vi "ActionVIOnRecompile.vi"(8 "error in":errorcluster, 9 "Timeout (ms)":u32, 10 "Runtime Configurable Section Path":string, 11 "Device Item Ref in":T1 format="%.0x") -> (0 "error out":errorcluster)   [LabVIEW 2026, in "Runtime Configuration Support Inline Async Example Custom Device System Explorer.lvlib"]
uses:
  Runtime Configuration Support Inline Async Example Custom Device System Explorer.lvlib
  <vilib>/NI VeriStand/Custom Device API/Custom Device Item Ref.ctl
  <vilib>/NI VeriStand/Custom Device API/Custom Device Channel Type.ctl
  <vilib>/NI VeriStand/Custom Device API/Block Data Reference.ctl
  <vilib>/NI VeriStand/Custom Device API/Data Reference.ctl
  Shared/Reconfigured.Settings.ctl
  Shared/Compiled.Settings.ctl
  <vilib>/NI VeriStand/Custom Device API/Get Item Property (I32).vi
  Error Constants.vi
  <vilib>/NI VeriStand/Custom Device API/Get Item Property (Variant).vi
  <vilib>/NI VeriStand/Execution/CustomDevice/NI VeriStand - Send Custom Device Message (Byte Array).vi
  <vilib>/NI VeriStand/Custom Device API/Custom Device API.lvlib
  <vilib>/NI/NIVS Inline Async API/_Data Access System Explorer/Data Access System Explorer.lvlib
  <vilib>/NI VeriStand/execution/CustomDevice/NI_VS Custom Device ExecutionAPI.lvlib
  Shared/Runtime Configuration Support Inline Async Example Custom Device Shared.lvlib
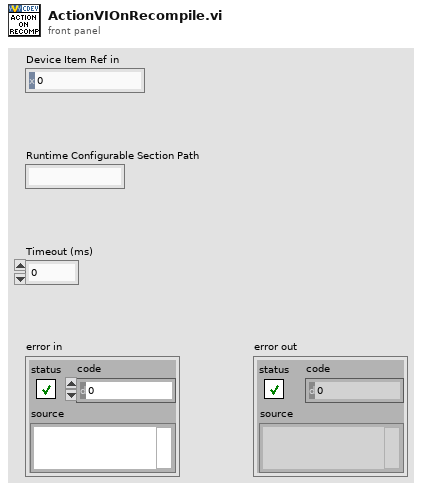
[diagram p1: front panel]
types:
  T1 = typedef "Custom Device API.lvlib/Custom Device Item Ref.ctl" = u64
  T2 = typedef "Runtime Configuration Support Inline Async Example Custom Device Shared.lvlib/Reconfigured.Settings.ctl" = cluster{"Compiled.Settings":T3, "Compiled Inline Async Settings":cluster{"Read":cluster{"Refs":T4[], "Values":dbl[]}[], "Write":cluster{"Refs":T4[], "Values":dbl[]}[], "ReadWrite":cluster{"Refs":T5[], "Values":dbl[], "Reset Values":dbl[]}[], "LUT":variant}, "Response Ref":refnum<queue>}
  T3 = typedef "Runtime Configuration Support Inline Async Example Custom Device Shared.lvlib/Compiled.Settings.ctl" = cluster{"Name":string, "Async Init Timeout":u16, "Inport SignalIDs":i32[], "Outport SignalIDs":i32[], "Inport Values":dbl[], "Outport Values":dbl[], "Dynamic Config Status":bool, "Device Error":errorcluster}
  T4 = typedef "Custom Device API.lvlib/Block Data Reference.ctl" = cluster{"Data Reference":T5, "Offset":u64, "Length":u64}
  T5 = typedef "Custom Device API.lvlib/Data Reference.ctl" = i32
  T6 = typedef "Custom Device API.lvlib/Custom Device Channel Type.ctl" = enum16{"Input", "Output"}
  T7 = cluster{"Name":string, "Type":enum16{"Output/Write", "Input/Read", "Input/ReadWrite"}, "VS Refs":T1[]}
  T8 = enum16{"Output/Write", "Input/Read", "Input/ReadWrite"}
  T9 = cluster{"Read":cluster{"Refs":T4[], "Values":dbl[]}[], "Write":cluster{"Refs":T4[], "Values":dbl[]}[], "ReadWrite":cluster{"Refs":T5[], "Values":dbl[], "Reset Values":dbl[]}[], "LUT":variant}
  T10 = typedef "Custom Device API.lvlib/Custom Device Item Info.ctl" = cluster{"Name":string, "Is Channel":bool, "GUID":string, "Is Waveform":bool}
  T11 = cluster{"Name":string, "Type":enum16{"Output/Write", "Input/Read", "Input/ReadWrite"}, "VS Refs":T1[]}[]
  T12 = typedef "NI_VS Custom Device ExecutionAPI.lvlib/Custom Device Ref.ctl" = refnum<k24>
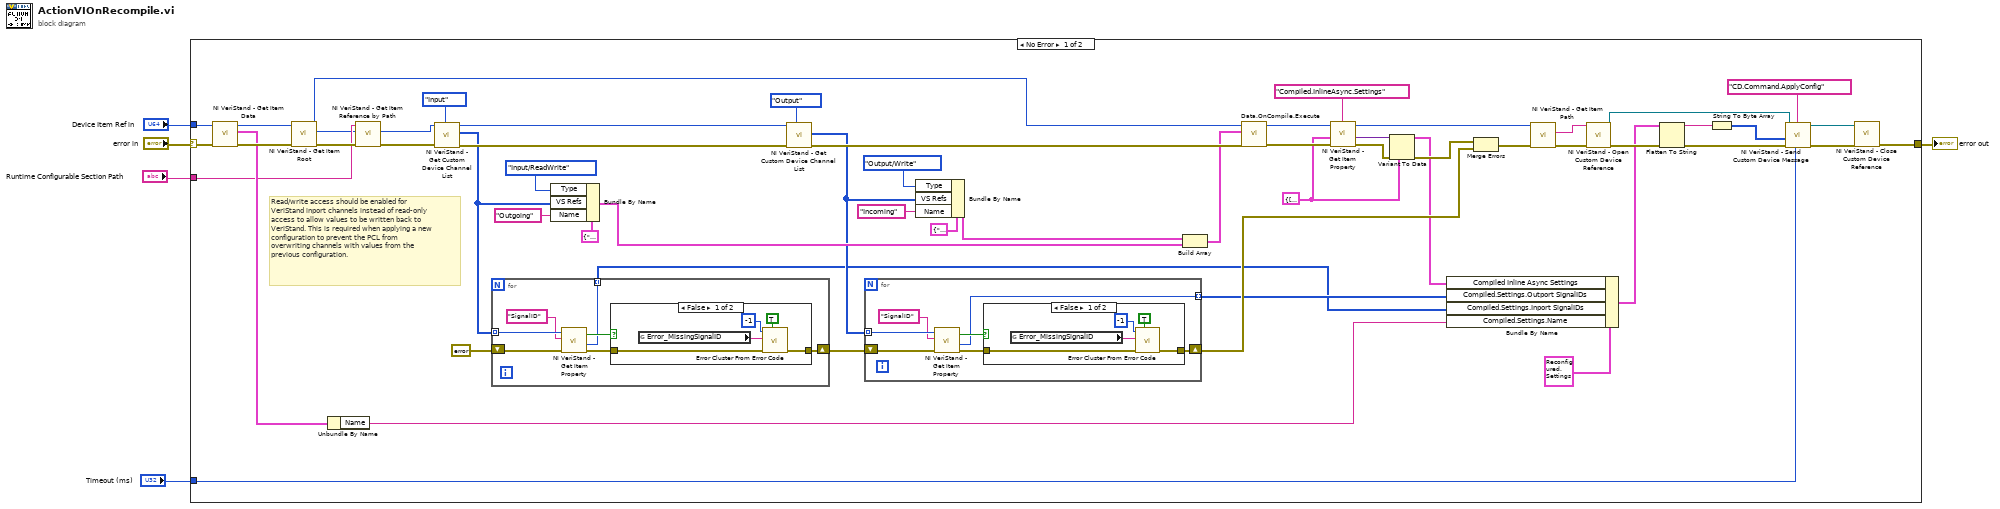
[diagram p0: block diagram]
diagram:
  n1 = case shown="No Error" "error in" {
    selector: "error in" -> [w62 w89]
    tunnel: [w54 w89] -> w4
    tunnel: "Device Item Ref in" -> [w44 _]
    tunnel: "Runtime Configurable Section Path" -> [w32 _]
    tunnel: "Timeout (ms)" -> [w17 _]
    frame No Error {
      w15 = T9 {"Read"=[], "Write"=[], "ReadWrite"=[], "LUT"=variant} ("Compiled.InlineAsync.Settings")
      # "Read/write access should be enabled for VeriStand inport channels instead of read-only access to allow values to be written back to VeriStand. This is required when applying a new configuration to prevent the PCL from overwriting channels with values from the previous configuration."
      n2 = call <vilib>:"NI VeriStand - Get Item Data.vi"("error in (no error)"=w62, "Item Ref in"=w44) -> ("error out"=w46:errorcluster, "Item Info"=w43:T10, "Item Ref out"=w8:T1)  [unwired: 6 in, 1 out]
      n3 = call <vilib>:"NI VeriStand - Get Item Root.vi"("error in (no error)"=w46, "Item Ref in"=w8) -> ("error out"=w45:errorcluster, "Root Ref out"=w9:T1, "Item Ref out"=w7:T1)  [unwired: 6 in, 1 out]
      n4 = Unbundle By Name(w43) -> ("Name"=w42:string)
      n5 = call <vilib>:"NI VeriStand - Get Item Reference by Path.vi"("error in (no error)"=w45, "Root Ref"=w9, "Item Path in"=w32) -> ("error out"=w61:errorcluster, "Item Ref"=w31:T1)  [unwired: 5 in, 2 out]
      n6 = call <vilib>:"NI VeriStand - Get Custom Device Channel List.vi"("Channel Type"=Custom_Device_Channel_Type."Input", "error in (no error)"=w61, "Device Ref in"=w31) -> ("error out"=w60:errorcluster, "Specified Channel Ref List"=w14:T1[], "Device Ref out"=w28:T1)  [unwired: 6 in]
      n7 = for {
        tunnel: w14 -> [w79] mode=indexing
        shift-right: [w81] -> w50
        shift-left: errorcluster {"status"=FALSE, "code"=0, "source"=""} ("error out") -> [w80]
        tunnel: [w76] -> w10 mode=indexing
        n8 = call-poly <vilib>:"NI VeriStand - Get Item Property.vi"("error in (no error)"=w80, "Property Name"="SignalID", "Item Ref in"=w79) -> ("error out"=w82:errorcluster, "Value"=w76:i32, "Found?"=w77:bool)  [unwired: 5 in, 1 out]
        n9 = case shown="False" w77 {
          tunnel: w82 -> [w87 w88]
          tunnel: [w86 w88] -> w81
          frame False {
            n10 = global read "Error Constants.vi" "Error_MissingSignalID"() -> (w84:string)
            n11 = call <vilib>:"Error Cluster From Error Code.vi"("show call chain? (False)"=TRUE, "error in (no error)"=w87, "error message (\"\")"=w84, "error code (0)"=-1) -> ("error out"=w86:errorcluster)  [unwired: 5 in]
          }
          frame True {
          }
        }
      }
      n12 = Bundle By Name(cluster=T7 {"Name"="", "Type"=enum."Output/Write", "VS Refs"=[]} ("Group"), "Type"=T8."Input/ReadWrite", "VS Refs"=w14, "Name"="Outgoing" ("Item Name")) -> (w33:T7)
      n13 = call <vilib>:"NI VeriStand - Get Custom Device Channel List.vi"("Channel Type"=Custom_Device_Channel_Type."Output", "error in (no error)"=w60, "Device Ref in"=w28) -> ("error out"=w59:errorcluster, "Specified Channel Ref List"=w13:T1[])  [unwired: 6 in, 1 out]
      n14 = for {
        tunnel: w13 -> [w66] mode=indexing
        shift-right: [w68] -> w47
        shift-left: w50 -> [w67]
        tunnel: [w63] -> w11 mode=indexing
        n15 = call-poly <vilib>:"NI VeriStand - Get Item Property.vi"("error in (no error)"=w67, "Property Name"="SignalID", "Item Ref in"=w66) -> ("error out"=w69:errorcluster, "Value"=w63:i32, "Found?"=w64:bool)  [unwired: 5 in, 1 out]
        n16 = case shown="False" w64 {
          tunnel: w69 -> [w74 w75]
          tunnel: [w73 w75] -> w68
          frame False {
            n17 = global read "Error Constants.vi" "Error_MissingSignalID"() -> (w71:string)
            n18 = call <vilib>:"Error Cluster From Error Code.vi"("show call chain? (False)"=TRUE, "error in (no error)"=w74, "error message (\"\")"=w71, "error code (0)"=-1) -> ("error out"=w73:errorcluster)  [unwired: 5 in]
          }
          frame True {
          }
        }
      }
      n19 = Bundle By Name(cluster=T7 {"Name"="", "Type"=enum."Output/Write", "VS Refs"=[]} ("Group"), "Type"=T8."Output/Write", "VS Refs"=w13, "Name"="Incoming" ("Item Name")) -> (w38:T7)
      n20 = Build Array(w38, w33) -> (w36:T11)
      n21 = call <vilib>:"Data.OnCompile.Execute.vi"("error in"=w59, "VS Ref Groups"=w36, "Custom Device Ref"=w7) -> ("error out"=w57:errorcluster, "Custom Device Ref"=w24:T1)  [unwired: 7 in]
      n22 = call-poly <vilib>:"NI VeriStand - Get Item Property.vi"("error in (no error)"=w57, "Default Value"=w15, "Property Name"="Compiled.InlineAsync.Settings", "Item Ref in"=w24) -> ("error out"=w52:errorcluster, "Value"=w22:variant, "Item Ref out"=w16:T1)  [unwired: 4 in, 1 out]
      n23 = Variant To Data(error in=w52, type=w15, Variant=w22) -> (data=w12:T9, error out=w49:errorcluster)
      n24 = Bundle By Name(cluster=T2 {"Compiled.Settings"={"Name"="", "Async Init Timeout"=0, "Inport SignalIDs"=[], "Outport SignalIDs"=[], "Inport Values"=[], "Outport Values"=[], "Dynamic Config Status"=FALSE, "Device Error"={"status"=FALSE, "code"=0, "source"=""}}, "Compiled Inline Async Settings"={"Read"=[], "Write"=[], "ReadWrite"=[], "LUT"=variant}, "Response Ref"=refnum} ("ReConfigured.Settings"), "Compiled Inline Async Settings"=w12, "Compiled.Settings.Outport SignalIDs"=w11, "Compiled.Settings.Inport SignalIDs"=w10, "Compiled.Settings.Name"=w42) -> (w21:T2)
      n25 = Merge Errors(w49, w47) -> (w48:errorcluster)
      n26 = call <vilib>:"NI VeriStand - Get Item Path.vi"("error in (no error)"=w48, "Item Ref in"=w16) -> ("error out"=w58:errorcluster, "Path"=w27:string)  [unwired: 6 in, 2 out]
      n27 = call <vilib>:"NI VeriStand - Open Custom Device Reference.vi"("error in (no error)"=w58, "Custom Device Path"=w27) -> ("error out"=w56:errorcluster, "Custom Device"=w26:T12)  [unwired: 8 in]
      n28 = Flatten To String(anything=w21, error in (no error)=w56) -> (data string=w20:string, error out=w55:errorcluster)  [unwired: 2 in, 1 out]
      n29 = String To Byte Array(string=w20) -> (unsigned byte array=w19:u8[])
      n30 = call-poly <vilib>:"NI VeriStand - Send Custom Device Message.vi"("Timeout ms (5000)"=w17, "error in (no error)"=w55, "Data"=w19, "Command"="CD.Command.ApplyConfig", "Custom Device in"=w26) -> ("error out"=w53:errorcluster, "Custom Device out"=w18:T12)  [unwired: 4 in, 1 out]
      n31 = call <vilib>:"NI VeriStand - Close Custom Device Reference.vi"("error in (no error)"=w53, "Custom Device"=w18) -> ("error out"=w54:errorcluster)  [unwired: 9 in]
    }
    frame Error {
    }
  }
  "error out" <- w4
